vi "PiezoAndSnapshot.vi"() -> ()   [LabVIEW 2013]
doc: "v4: Added NI DAQ board instead of LabJack\n\nv5: Modified autofocus routine. Changed to triangle wave - AUTOFOCUS DOES NOT WORK ANYMORE\n\nv6: Modified autofocus to work with Triangle Wave. Added Saved Image Number to Lab Jack String."
uses:
  <vilib>/Platform/TimedLoop/XDataNode/timing_clust.ctl
  <vilib>/Platform/TimedLoop/XDataNode/nitl_modes.ctl
  <vilib>/Platform/TimedLoop/XDataNode/wakeup.ctl
  <vilib>/event_ctls.llb/eventvkey.ctl
  <vilib>/DAQmx/read.llb/DAQmx Read (Analog 1D DBL NChan 1Samp).vi
  <vilib>/DAQmx/miscellaneous.llb/DAQmx Fill In Error Info.vi
  <vilib>/platform/TimedLoop/XDataNode/XDataNode.xnode
  <vilib>/Platform/TimedLoop/XDataNode/XDNodeRunTimeDep.lvlib
panel:
  out "Voltage offset":dbl
  in  "Micron offset":dbl
  out "Counter":string
  out "TiffPath":string
  in  "Snap?":bool
  out "Stage Y":i32=31604
  out "Stage X":i32=-158372
  out "TotalFramesHidden":i32=27980
  out "Saved Images Hidden":i32=786
  out "sCMOS Image":u16[][](graph)
  in  "ROI":T1={"Horizontal Offset"=424, "Vertical Offset"=558, "Horizontal Width"=1200, "Vertical Width"=600}
  in  "Exposure (ms)":dbl=5.0
  in  "Binning":u16(ring)=1 items=["1x1"=1, "2x2"=2, "4x4"=4]
  out "Written":string="\r\r---------------------  NEW FILE  ---------------------\rO:\\20141210\\BrainScanner20141210_124111\r\r12/10/2014 12:42 PM\rcalib1\n\r\r12/10/2014 12:42 PM\rcalib 2\n\r\r12/10/2014 12:43 PM\rcalib 3\n\r\r"
  in  "Comments":string
  out "User Comments  File":path=path "O:/20141210/Comments.txt"
  out "Quit Pushed?":bool=TRUE
  out "Camera Trigger":dbl=0.00885779825410911 format="%.6f"
  out "Camera Frame File":path=path "O:/20141210/BrainScanner20141210_124111/CameraFrameData.txt"
  out "FxnGen Sync":dbl=3.893227260535598 format="%.6f"
  out "Z Sensor":dbl=0.9636767585825825 format="%.6f"
  out "LabJack File":path=path "O:/20141210/BrainScanner20141210_124111/LabJackData.txt"
  out "Current Image":u16[][](array[numeric])
  out "FuncGen Voltage":dbl=0.9652874538141194 format="%.6f"
  out "Z-ramp DC Offset":dbl=1.0
  out "sCMOS Camera Image File":path=path "O:/20141210/BrainScanner20141210_124111/sCMOS_Frames_U16_1024x1024.dat"
  out "Save Directory":path=path "O:/20141210/BrainScanner20141210_124111"
  out "Camera Info":string="C11440-22C; S/N: 751007; 2.50.A"
  in  "Quit":bool
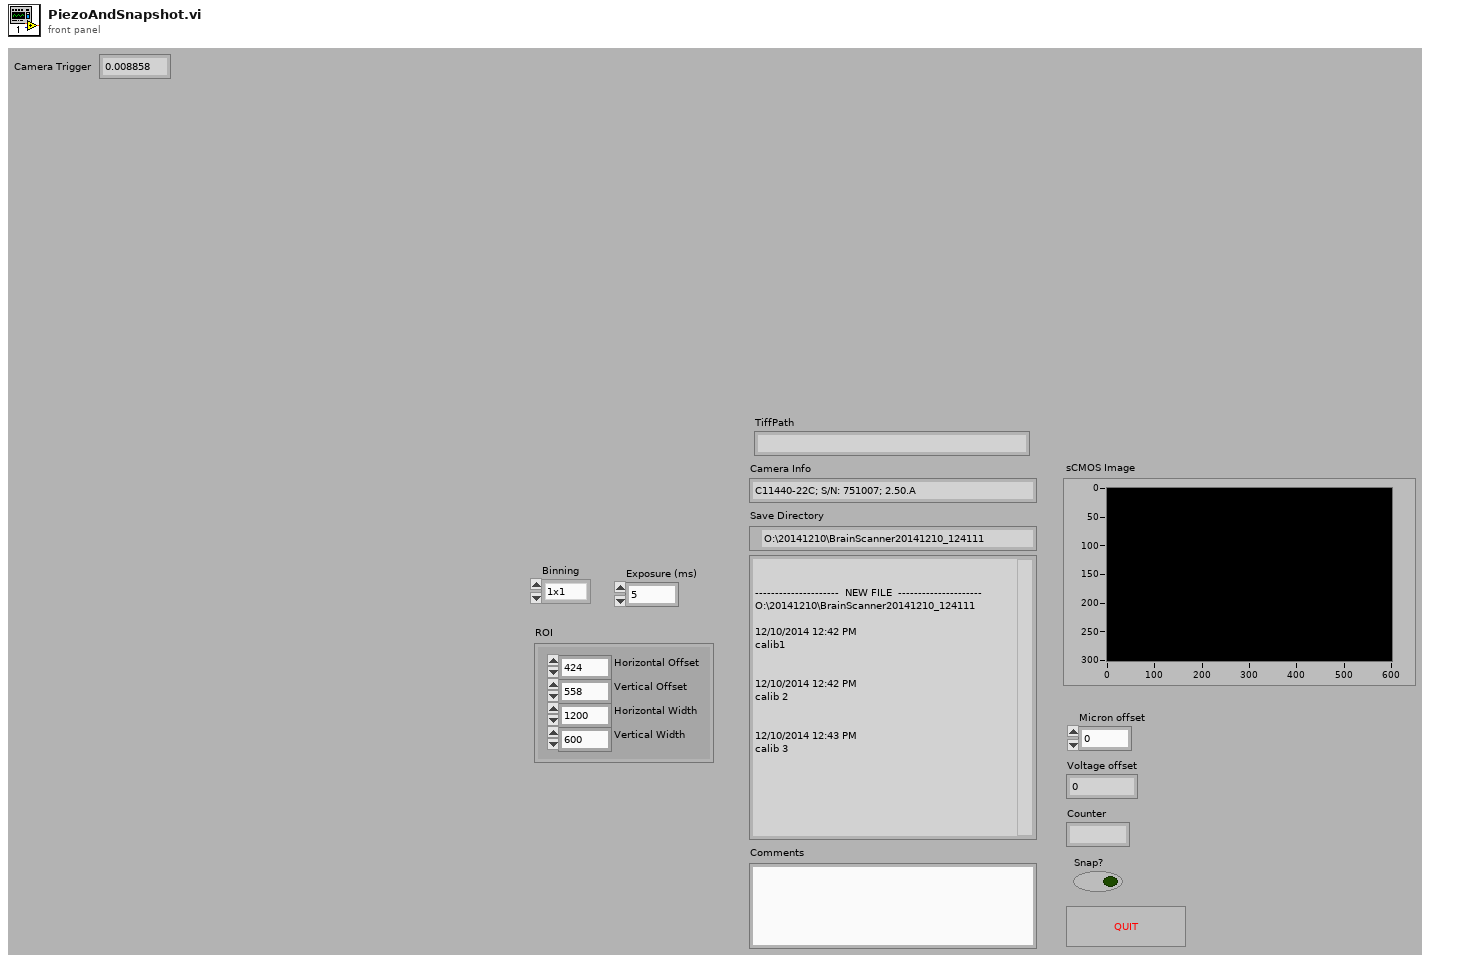
[diagram p1: front panel]
types:
  T1 = cluster{"Horizontal Offset":i32, "Vertical Offset":i32, "Horizontal Width":i32, "Vertical Width":i32}
  T2 = enum16{"open", "replace", "create", "open or create", "replace or create", "replace or create with confirmation"}
  T3 = cluster{"height":u32, "width":u32, "datatype":u32}
  T4 = cluster{"Mode":u32, "Polarity":u32, "Period":dbl, "Delay":dbl}
  T5 = typedef "XDNodeRunTimeDep.lvlib/timing_clust.ctl" = cluster{"Expected End [f-1]":u64, "Actual End [f-1]":u64, "Finished Late? [f-1]":bool, "Expected End [i-1]":u64, "Actual End [i-1]":u64, "Finished Late? [i-1]":bool, "Expected Start [i]":u64, "Actual Start [i]":u64, "Expected Start [f]":u64, "Actual Start [f]":u64, "Source Name":string, "Structure Name":string, "Period":i64, "Deadline":i64, "Offset":i64, "Start":i64, "Priority":i32, "Timeout":i32, "Mode":T6, "Wakeup Reason":T7, "Error":errorcluster, "Source Type":string, "Secondary Source Type":string, "Global End Time":u64, "Global Start Time":u64, "Frame Duration":u64, "Iteration Duration":u64, "Assigned CPU":i32, "I/O Scan Engine Mode":u32}
  T6 = typedef "XDNodeRunTimeDep.lvlib/nitl_modes.ctl" = enum32{"No Change", "Process missed periods, maintain original phase", "Discard missed periods, maintain original phase", "Process missed periods, ignore original phase", "Discard missed periods, ignore original phase"}
  T7 = typedef "XDNodeRunTimeDep.lvlib/wakeup.ctl" = enum32{"Normal", "Aborted", "Asynchronous wakeup", "Timing source error", "Timed loop error", "Timeout"}
  T8 = typedef "eventvkey.ctl" = enum16{"ASCII", "Enter", "Return", "Shift", "Ctrl", "Alt", "Cmd", "Opt", "Caps", "NumLock", "Clear", "Break", "Up", "Down", "Left", "Right", "Insert", "Delete", "Home", "End", "PageUp", "PageDown", "Escape", "Help", "Pause", "ScrollLock", "F1", "F2", "F3", "F4", "F5", "F6", "F7", "F8", "F9", "F10", "F11", "F12", "F13", "F14", "F15", "F16", "F17", "F18", "F19", "F20", "F21", "F22", "F23", "F24", "Play", "VolumeUp", "VolumeDown", "Mute", "Two Byte Char"}
  T9 = typedef "IMAQ Image.ctl" = refnum<image>
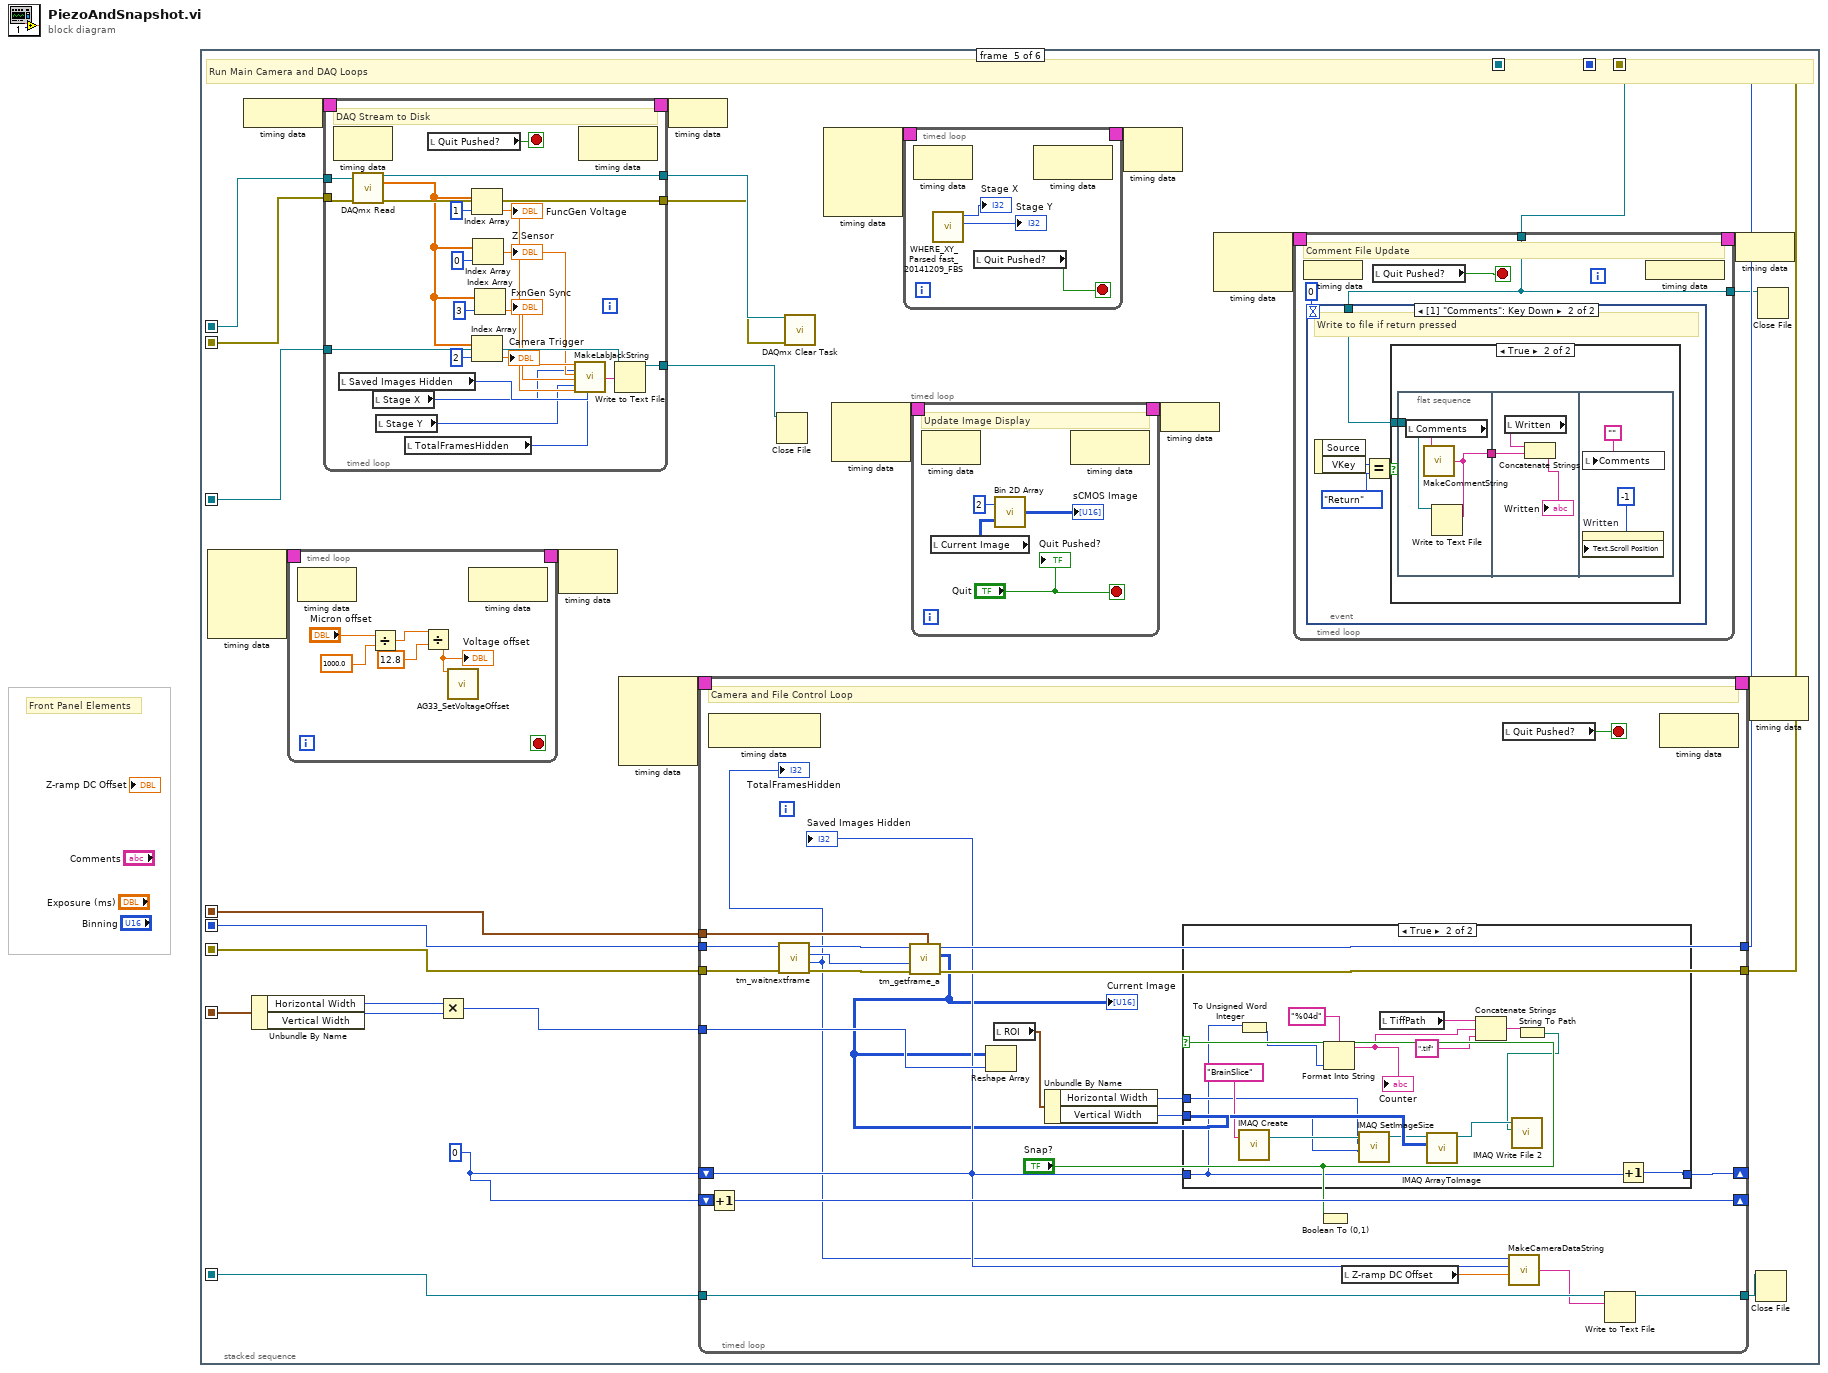
[diagram p0: block diagram]
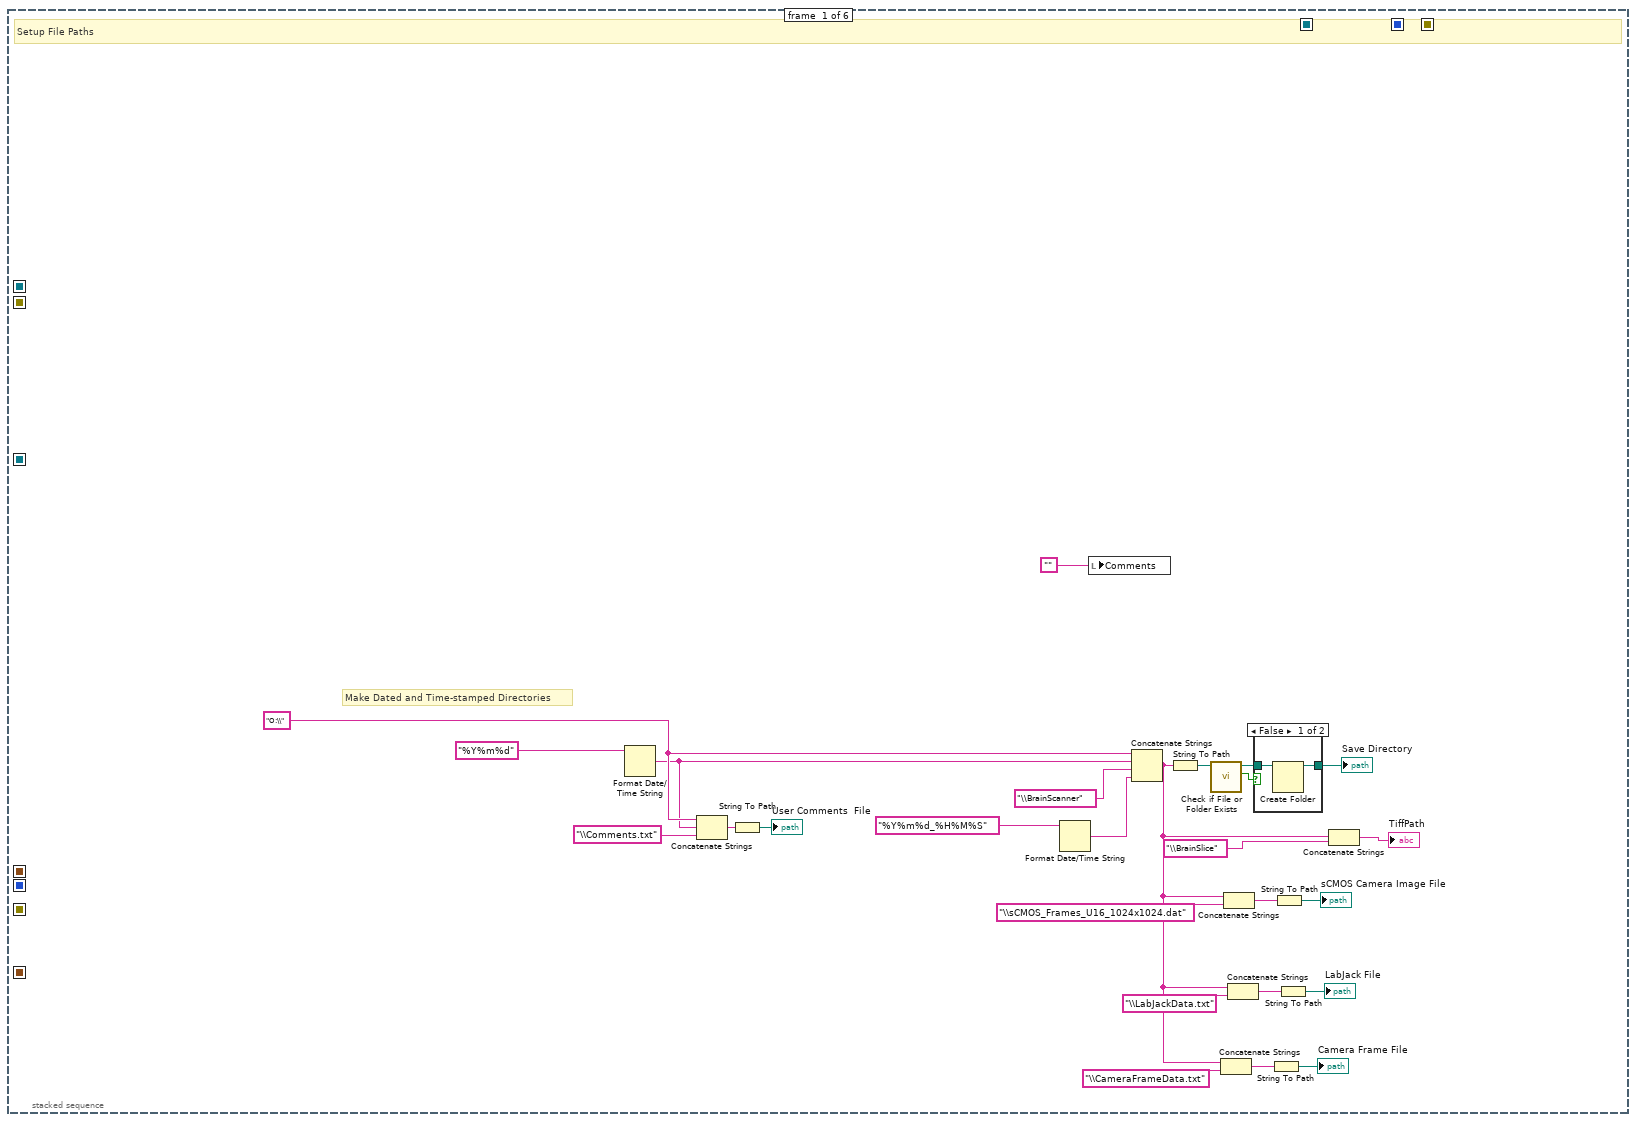
[diagram p2: hidden frame]
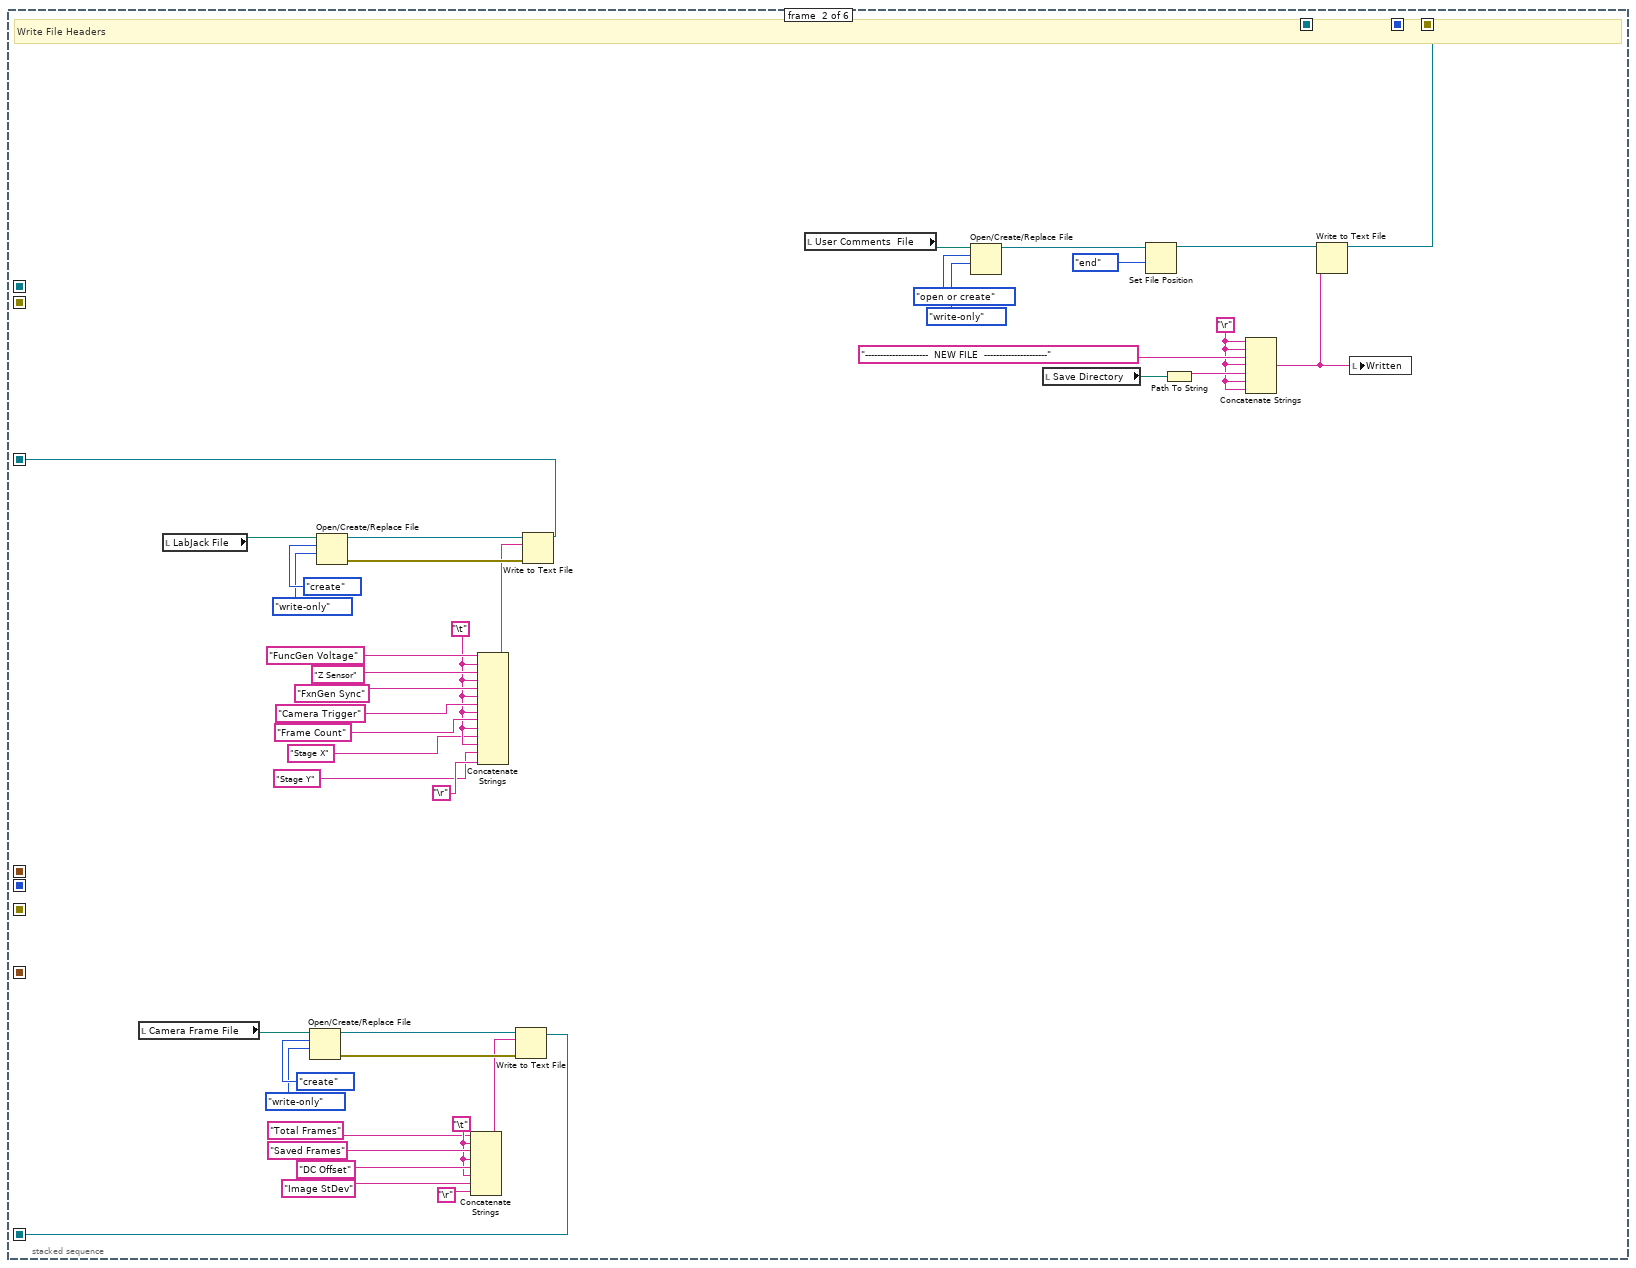
[diagram p4: hidden frame]
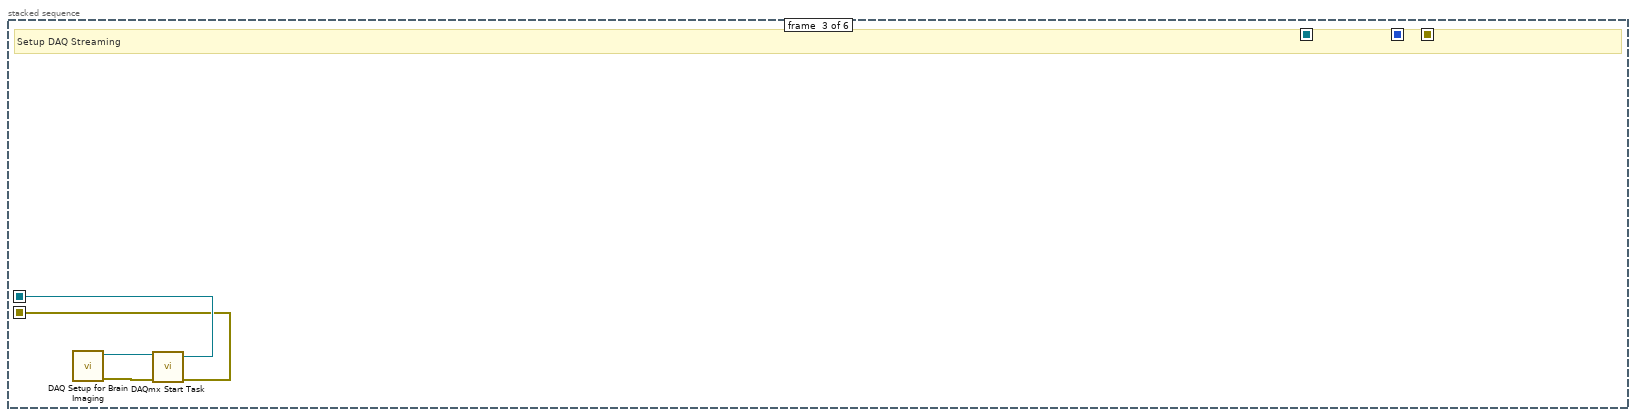
[diagram p5: hidden frame]
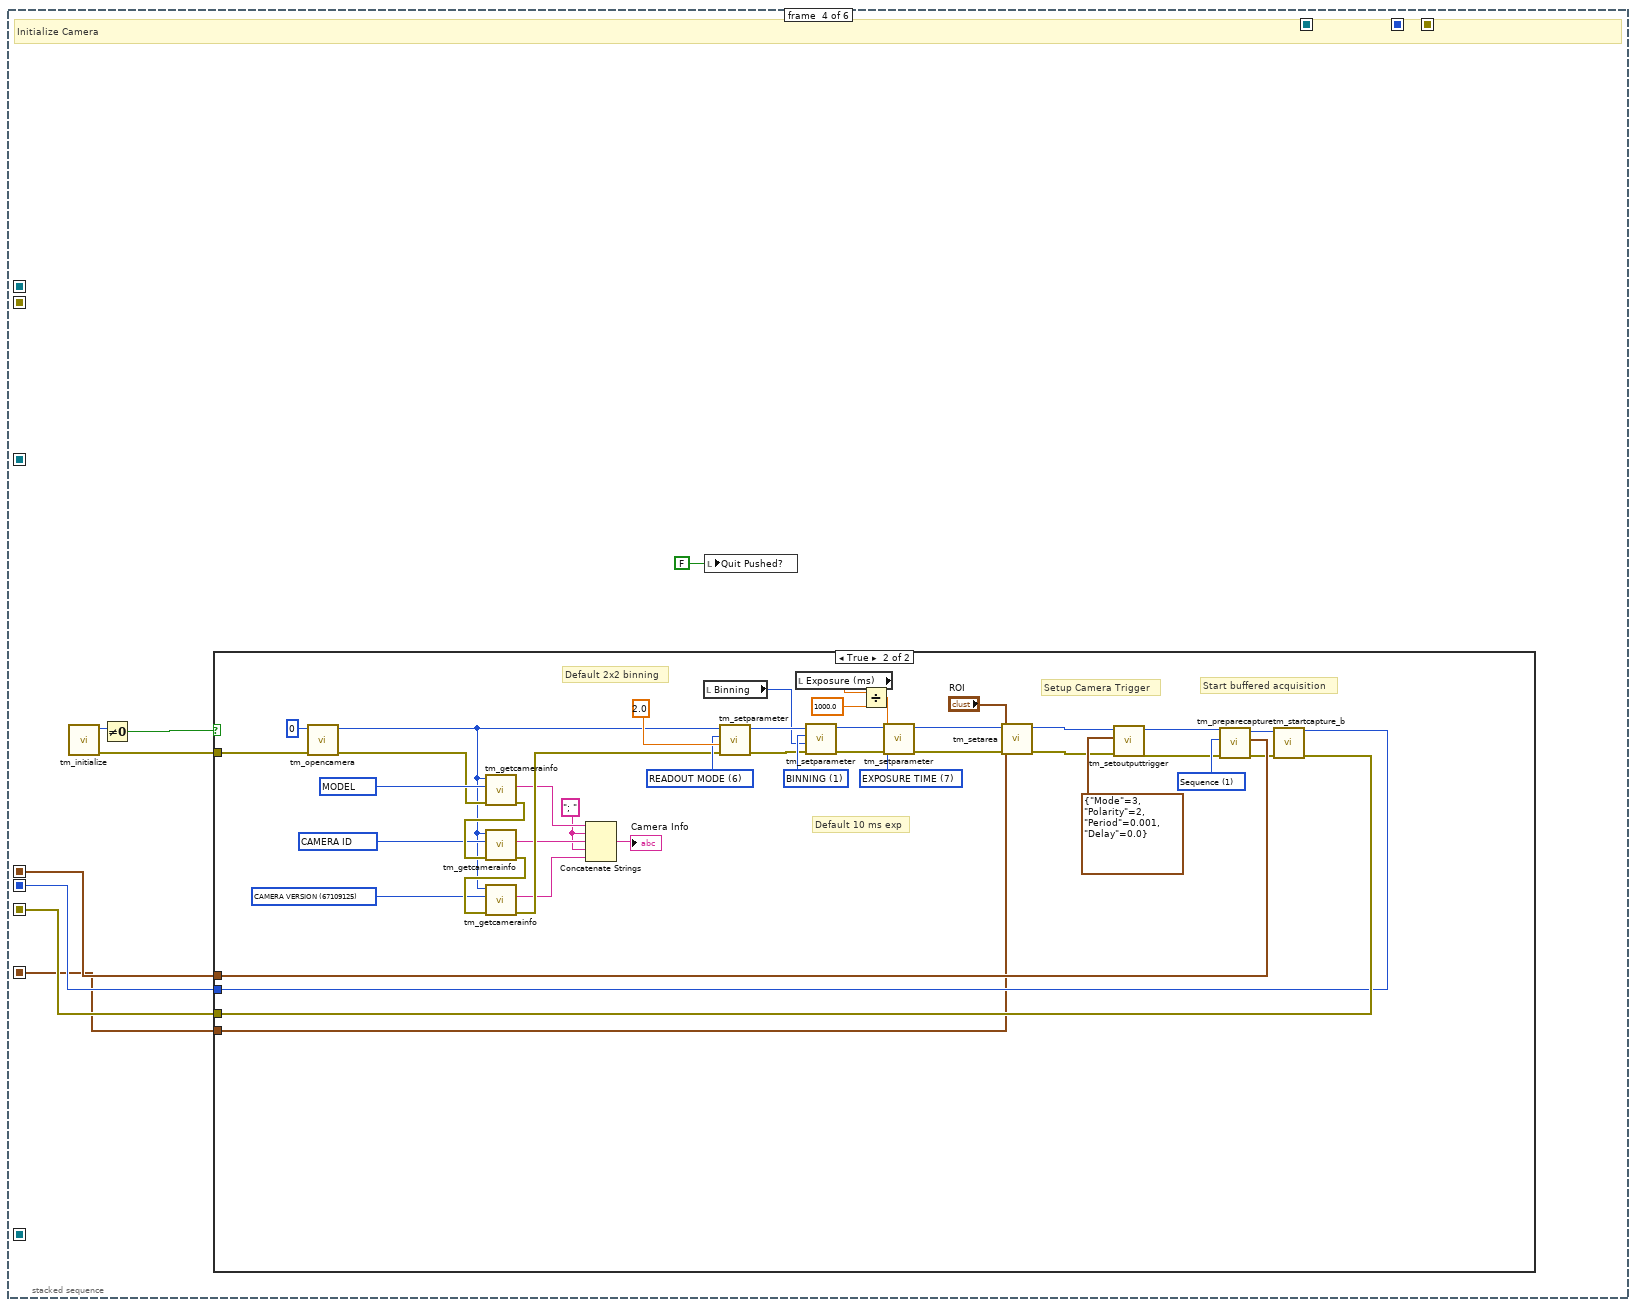
[diagram p6: hidden frame]
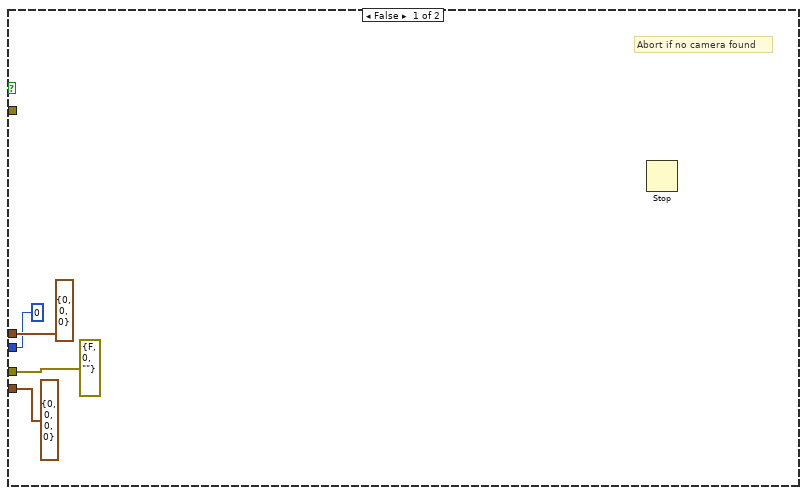
[diagram p7: hidden frame]
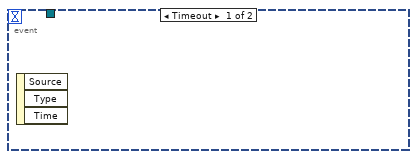
[diagram p8: hidden frame]
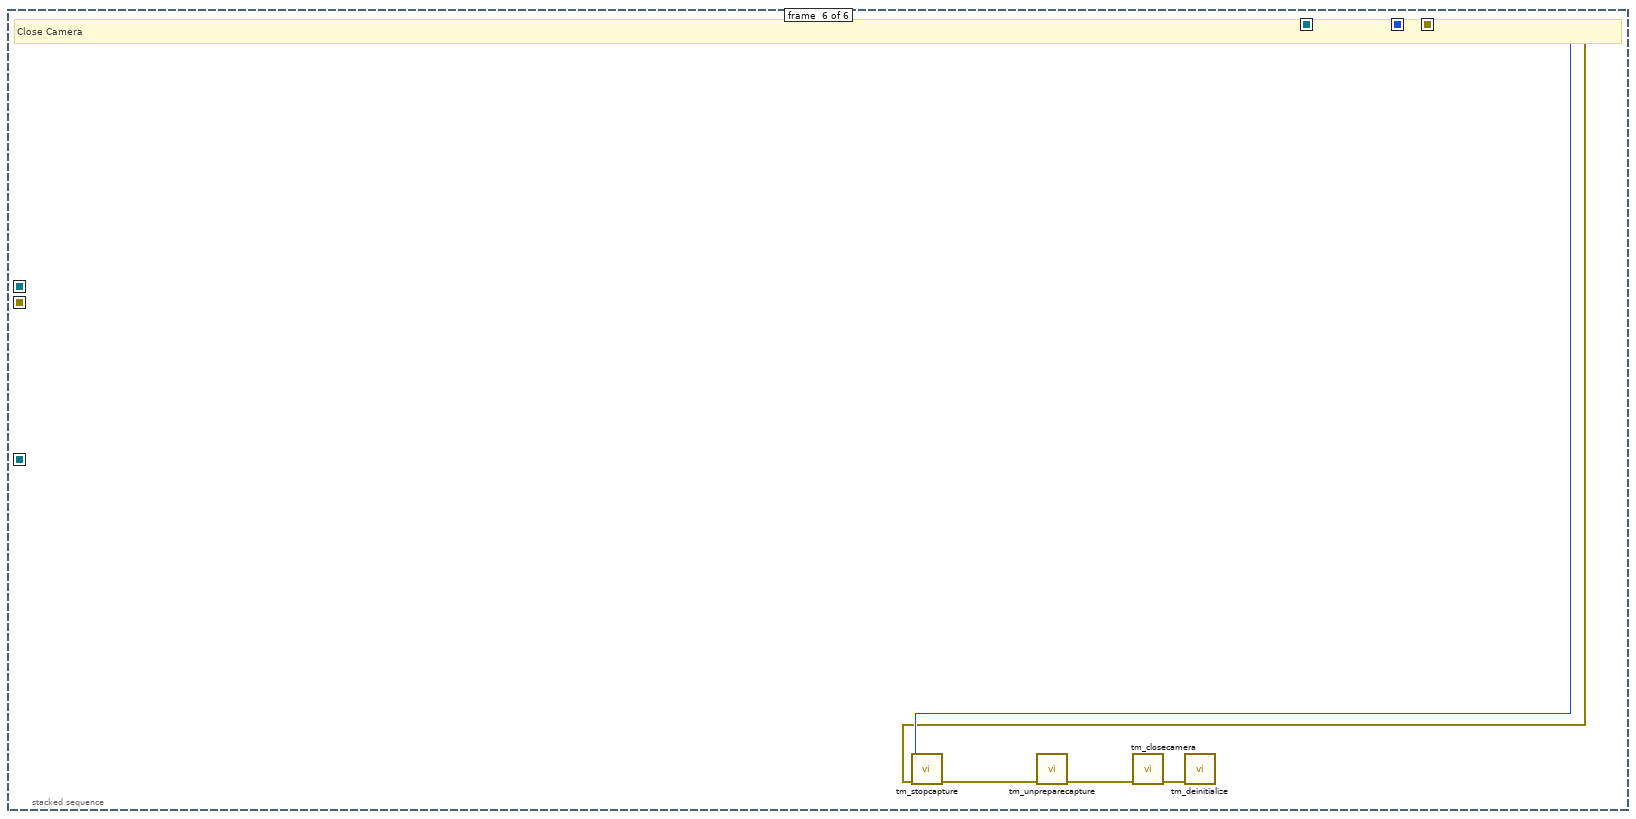
[diagram p11: hidden frame]
diagram:
  # "Front Panel Elements"
  n1 = stacked-sequence {
    seq-local: [_ _ _ w77 _ _] -> [_ _ _ _ w156 _]
    seq-local: [_ _ _ w78 _ _] -> [_ _ _ _ w159 _]
    seq-local: [_ _ _ w79 _ _] -> [_ _ _ _ w155 _]
    seq-local: [_ _ _ _ w158 _] -> [_ _ _ _ _ w276]
    seq-local: [_ _ _ _ w157 _] -> [_ _ _ _ _ w275]
    seq-local: [_ w64 _ _ _ _] -> [_ _ _ _ w147 _]
    seq-local: [_ _ w74 _ _ _] -> [_ _ _ _ w145 _]
    seq-local: [_ _ w73 _ _ _] -> [_ _ _ _ w146 _]
    seq-local: [_ w54 _ _ _ _] -> [_ _ _ _ w144 _]
    seq-local: [_ w42 _ _ _ _] -> [_ _ _ _ w140 _]
    seq-local: [_ _ _ w75 _ _] -> [_ _ _ _ w136 _]
    frame #0 {
      w7 = "O:\\"
      # "Make Dated and Time-stamped Directories"
      # "Setup File Paths"
      n2 = Format Date/Time String(time format string (%c)="%Y%m%d") -> (date/time string=w6:string)  [unwired: 2 in]
      n3 = Concatenate Strings(w7, w6, "\\Comments.txt" ("string")) -> (w4:string)
      n4 = String To Path(string=w4) -> (path=→"User Comments  File":path)
      n5 = Format Date/Time String(time format string (%c)="%Y%m%d_%H%M%S") -> (date/time string=w21:string)  [unwired: 2 in]
      n6 = local write "Comments"("") -> ()
      n7 = Concatenate Strings(w7, w6, "\\BrainScanner", w21) -> (w3:string)
      n8 = String To Path(string=w3) -> (path=w20:path)
      n9 = call <vilib>:"Check if File or Folder Exists.vi"("path"=w20) -> ("file or folder exists?"=w25:bool, "dup path"=w24:path)  [unwired: 8 in, 1 out]
      n10 = Concatenate Strings(w3, "\\CameraFrameData.txt" ("string")) -> (w12:string)
      n11 = Concatenate Strings(w3, "\\sCMOS_Frames_U16_1024x1024.dat" ("string")) -> (w17:string)
      n12 = Concatenate Strings(w3, "\\LabJackData.txt" ("string")) -> (w15:string)
      n13 = case shown="False" w25 {
        tunnel: [w27 w29] -> w19
        tunnel: w24 -> [w28 w29]
        frame False {
          n14 = Create Folder(path (use dialog)=w28) -> (created path=w27:path)  [unwired: 2 in, 2 out]
        }
        frame True {
        }
      }
      "Save Directory" <- w19
      n15 = String To Path(string=w12) -> (path=→"Camera Frame File":path)
      n16 = String To Path(string=w17) -> (path=→"sCMOS Camera Image File":path)
      n17 = String To Path(string=w15) -> (path=→"LabJack File":path)
      n18 = Concatenate Strings(w3, "\\BrainSlice" ("string")) -> (→"TiffPath":string)
    }
    frame #1 {
      w37 = "\r"
      w36 = "\t"
      w33 = "\t"
      # "Write File Headers"
      n19 = local read "Camera Frame File"() -> (w53:path)
      n20 = local read "LabJack File"() -> (w65:path)
      n21 = Open/Create/Replace File(file path (use dialog)=w53, operation (0:open)=T2."create", access (0:read/write)=enum16{"read/write", "read-only", "write-only"}."write-only") -> (refnum out=w63:refnum<file>, error out=w62:errorcluster)  [unwired: 3 in, 1 out]
      n22 = Open/Create/Replace File(file path (use dialog)=w65, operation (0:open)=T2."create", access (0:read/write)=enum16{"read/write", "read-only", "write-only"}."write-only") -> (refnum out=w70:refnum<file>, error out=w69:errorcluster)  [unwired: 3 in, 1 out]
      n23 = Concatenate Strings("Total Frames", w36, "Saved Frames", w36, "DC Offset", w36, "Image StDev", "\r") -> (w58:string)
      n24 = Concatenate Strings("FuncGen Voltage", w33, "Z Sensor", w33, "FxnGen Sync", w33, "Camera Trigger", w33, "Frame Count", w33, "Stage X" ("string"), w33, "Stage Y" ("string"), "\r") -> (w68:string)
      n25 = Write to Text File(file (use dialog)=w63, text=w58, error in=w62) -> (refnum out=w54:refnum<file>)  [unwired: 1 in, 2 out]
      n26 = Write to Text File(file (use dialog)=w70, text=w68, error in=w69) -> (refnum out=w64:refnum<file>)  [unwired: 1 in, 2 out]
      n27 = local read "User Comments  File"() -> (w48:path)
      n28 = Open/Create/Replace File(file path (use dialog)=w48, operation (0:open)=T2."open or create", access (0:read/write)=enum16{"read/write", "read-only", "write-only"}."write-only") -> (refnum out=w45:refnum<file>)  [unwired: 3 in, 2 out]
      n29 = local read "Save Directory"() -> (w40:path)
      n30 = Set File Position(refnum=w45, from (0:start)=enum16{"start", "end", "current"}."end") -> (refnum out=w43:refnum<file>)  [unwired: 2 in, 1 out]
      n31 = Path To String(path=w40) -> (string=w39:string)
      n32 = Concatenate Strings(w37, w37, "---------------------  NEW FILE  ---------------------", w37, w39, w37, w37) -> (w38:string)
      n33 = Write to Text File(file (use dialog)=w43, text=w38) -> (refnum out=w42:refnum<file>)  [unwired: 2 in, 2 out]
      n34 = local write "Written"(w38) -> ()
    }
    frame #2 {
      # "Setup DAQ Streaming"
      n35 = call "DAQ Setup for Brain Imaging.vi"() -> ("error out"=w71:errorcluster, "task out"=w72:refnum<k21>)  [unwired: 10 in]
      n36 = call <vilib>:"DAQmx Start Task.vi"("task/channels in"=w72, "error in"=w71) -> ("task out"=w74:refnum<k21>, "error out"=w73:errorcluster)  [unwired: 12 in]
    }
    frame #3 {
      # "Initialize Camera"
      n37 = call <userlib>:"tm_initialize.vi"() -> ("error out"=w82:errorcluster, "Number Of Cameras"=w80:u32)  [unwired: 10 in]
      n38 = Not Equal To 0?(x=w80) -> (x != 0?=w81:bool)
      n39 = case shown="True" w81 {
        tunnel: w82 -> [_ w127]
        tunnel: [errorcluster {"status"=FALSE, "code"=0, "source"=""} ("error out") w95] -> w79
        tunnel: [u32 0 ("Handle out") w94] -> w77
        tunnel: [T3 {"height"=0, "width"=0, "datatype"=0} ("Buffer Info") w116] -> w78
        tunnel: [T1 {"Horizontal Offset"=0, "Vertical Offset"=0, "Horizontal Width"=0, "Vertical Width"=0} ("ROI") "ROI"] -> w75
        frame False {
          # "Abort if no camera found"
          n40 = Stop() -> ()  [unwired: 1 in]
        }
        frame True {
          w100 = "; " ("string")
          w114 = u32 6 items=["BINNING"=1, "BITS PER CHANNEL"=2, "ACTIVE VIEW INDEX"=3, "CCD MODE"=4, "SENSOR MODE"=5, "READOUT MODE"=6, "EXPOSURE TIME"=7, "CONTRAST GAIN"=8, "CONTRAST OFFSET"=9, "LIGHT MODE"=10, "SENSITIVITY"=11, "WHITE BALANCE"=12, "PHOTON IMAGING MODE"=13, "HIGH DYNAMIC RANGE MODE"=14, "TRIGGER SOURCE"=15, "TRIGGER ACTIVE"=16, "TRIGGER MODE"=17, "TRIGGER POLARITY"=18, "TRIGGER GLOBAL EXPOSURE"=19, "FIRST TRIGGER BEHAVIOR"=20, "TRIGGER TIMES"=21, "OUTPUT TRIGGER POLARITY"=22, "OUTPUT TRIGGER DELAY"=23, "OUTPUT TRIGGER PERIOD"=24, "TEMPERATURE"=25, "TEMPERATURE TARGET"=26, "SENSOR COOLER FAN"=27, "MECHANICAL SHUTTER"=28, "BACK FOCUS POSITION"=29, "FRAMEBUNDLE MODE"=30, "FRAMEBUNDLE NUMBER"=31, "LINEBUNDLE HEIGHT"=32, "TRIGGER CONNECTOR"=33, "IMAGE PIXEL TYPE"=34, "OUTPUT TRIGGER KIND"=35, "READOUT DIRECTION"=36, "CHANNEL SYNC"=37] ("Parameter")
          w117 = 1 items=["Snap", "Sequence"] ("Capture mode")
          w118 = u32 7 items=["BINNING"=1, "BITS PER CHANNEL"=2, "ACTIVE VIEW INDEX"=3, "CCD MODE"=4, "SENSOR MODE"=5, "READOUT MODE"=6, "EXPOSURE TIME"=7, "CONTRAST GAIN"=8, "CONTRAST OFFSET"=9, "LIGHT MODE"=10, "SENSITIVITY"=11, "WHITE BALANCE"=12, "PHOTON IMAGING MODE"=13, "HIGH DYNAMIC RANGE MODE"=14, "TRIGGER SOURCE"=15, "TRIGGER ACTIVE"=16, "TRIGGER MODE"=17, "TRIGGER POLARITY"=18, "TRIGGER GLOBAL EXPOSURE"=19, "FIRST TRIGGER BEHAVIOR"=20, "TRIGGER TIMES"=21, "OUTPUT TRIGGER POLARITY"=22, "OUTPUT TRIGGER DELAY"=23, "OUTPUT TRIGGER PERIOD"=24, "TEMPERATURE"=25, "TEMPERATURE TARGET"=26, "SENSOR COOLER FAN"=27, "MECHANICAL SHUTTER"=28, "BACK FOCUS POSITION"=29, "FRAMEBUNDLE MODE"=30, "FRAMEBUNDLE NUMBER"=31, "LINEBUNDLE HEIGHT"=32, "TRIGGER CONNECTOR"=33, "IMAGE PIXEL TYPE"=34, "OUTPUT TRIGGER KIND"=35, "READOUT DIRECTION"=36, "CHANNEL SYNC"=37] ("Parameter")
          w119 = u32 1 items=["BINNING"=1, "BITS PER CHANNEL"=2, "ACTIVE VIEW INDEX"=3, "CCD MODE"=4, "SENSOR MODE"=5, "READOUT MODE"=6, "EXPOSURE TIME"=7, "CONTRAST GAIN"=8, "CONTRAST OFFSET"=9, "LIGHT MODE"=10, "SENSITIVITY"=11, "WHITE BALANCE"=12, "PHOTON IMAGING MODE"=13, "HIGH DYNAMIC RANGE MODE"=14, "TRIGGER SOURCE"=15, "TRIGGER ACTIVE"=16, "TRIGGER MODE"=17, "TRIGGER POLARITY"=18, "TRIGGER GLOBAL EXPOSURE"=19, "FIRST TRIGGER BEHAVIOR"=20, "TRIGGER TIMES"=21, "OUTPUT TRIGGER POLARITY"=22, "OUTPUT TRIGGER DELAY"=23, "OUTPUT TRIGGER PERIOD"=24, "TEMPERATURE"=25, "TEMPERATURE TARGET"=26, "SENSOR COOLER FAN"=27, "MECHANICAL SHUTTER"=28, "BACK FOCUS POSITION"=29, "FRAMEBUNDLE MODE"=30, "FRAMEBUNDLE NUMBER"=31, "LINEBUNDLE HEIGHT"=32, "TRIGGER CONNECTOR"=33, "IMAGE PIXEL TYPE"=34, "OUTPUT TRIGGER KIND"=35, "READOUT DIRECTION"=36, "CHANNEL SYNC"=37] ("Parameter")
          w120 = u32 67109122 items=["BUS"=67109121, "CAMERA ID"=67109122, "VENDOR"=67109123, "MODEL"=67109124, "CAMERA VERSION"=67109125, "DRIVER VERSION"=67109126, "MODULE VERSIOIN"=67109127, "DCAMAPI VERSION"=67109128] ("Info ID")
          w122 = u32 67109125 items=["BUS"=67109121, "CAMERA"=67109122, "VENDOR"=67109123, "MODEL"=67109124, "CAMERA VERSION"=67109125, "DRIVER VERSION"=67109126, "MODULE VERSIOIN"=67109127, "DCAMAPI VERSION"=67109128] ("Info ID")
          w125 = u32 67109124 items=["BUS"=67109121, "CAMERA"=67109122, "VENDOR"=67109123, "MODEL"=67109124, "CAMERA VERSION"=67109125, "DRIVER VERSION"=67109126, "MODULE VERSIOIN"=67109127, "DCAMAPI VERSION"=67109128] ("Info ID")
          # "Start buffered acquisition"
          # "Setup Camera Trigger"
          # "Default 10 ms exp"
          # "Default 2x2 binning"
          n41 = call <userlib>:"tm_opencamera.vi"("error in (no error)"=w127, "Camera Index"=u32 0) -> ("error out"=w121:errorcluster, "Handle out"=w106:u32)  [unwired: 8 in]
          n42 = call <userlib>:"tm_getcamerainfo.vi"("error in (no error)"=w121, "Info ID"=w125, "Handle in"=w106) -> ("error out"=w124:errorcluster, "String"=w103:string)  [unwired: 6 in, 1 out]
          n43 = call <userlib>:"tm_getcamerainfo.vi"("error in (no error)"=w124, "Info ID"=w120, "Handle in"=w106) -> ("error out"=w123:errorcluster, "String"=w102:string)  [unwired: 6 in, 1 out]
          n44 = call <userlib>:"tm_getcamerainfo.vi"("error in (no error)"=w123, "Info ID"=w122, "Handle in"=w106) -> ("error out"=w105:errorcluster, "String"=w101:string)  [unwired: 6 in, 1 out]
          n45 = Concatenate Strings(w103, w100, w102, w100, w101) -> (→"Camera Info":string)
          n46 = local read "Binning"() -> (w97:u16)
          n47 = call <userlib>:"tm_setparameter.vi"("error in (no error)"=w105, "Value in"=2.0, "Parameter"=w114, "Handle in"=w106) -> ("error out"=w107:errorcluster, "Handle out"=w108:u32)  [unwired: 6 in]
          n48 = local read "Exposure (ms)"() -> (w96:dbl)
          n49 = call <userlib>:"tm_setparameter.vi"("error in (no error)"=w107, "Value in"=w97, "Parameter"=w119, "Handle in"=w108) -> ("error out"=w112:errorcluster, "Handle out"=w113:u32)  [unwired: 6 in]
          n50 = Divide(x=w96, y=1000.0) -> (x/y=w98:dbl)
          n51 = call <userlib>:"tm_setparameter.vi"("error in (no error)"=w112, "Value in"=w98, "Parameter"=w118, "Handle in"=w113) -> ("error out"=w93:errorcluster, "Handle out"=w92:u32)  [unwired: 6 in]
          n52 = call <userlib>:"tm_setarea.vi"("error in (no error)"=w93, "Sub Region"="ROI", "Handle in"=w92) -> ("error out"=w90:errorcluster, "Handle out"=w91:u32)  [unwired: 7 in]
          n53 = call <userlib>:"tm_setoutputtrigger.vi"("error in (no error)"=w90, "Parameters"=T4 {"Mode"=3, "Polarity"=2, "Period"=0.001, "Delay"=0.0}, "Handle in"=w91) -> ("error out"=w88:errorcluster, "Handle out"=w89:u32)  [unwired: 7 in]
          n54 = call <userlib>:"tm_preparecapture.vi"("error in (no error)"=w88, "Capture mode"=w117, "Handle in"=w89) -> ("error out"=w110:errorcluster, "Buffer Info"=w116:T3, "Handle out"=w111:u32)  [unwired: 5 in, 1 out]
          n55 = call <userlib>:"tm_startcapture_b.vi"("error in (no error)"=w110, "Handle in"=w111) -> ("error out"=w95:errorcluster, "Handle out"=w94:u32)  [unwired: 8 in]
        }
      }
      n56 = local write "Quit Pushed?"(FALSE ("stop")) -> ()
    }
    frame #4 {
      w138 = 0
      # "Run Main Camera and DAQ Loops"
      n57 = node-c288() -> (w129:T5)  [unwired: 4 in]
      n58 = node-c288() -> (w152:T5)
      n59 = Unbundle By Name(w136) -> ("Horizontal Width"=w135:i32, "Vertical Width"=w134:i32)
      n60 = timed-loop {
        timing: w129 -> [_]
        timing-out: [_] -> w128
        stop <- _ stop-if-true
        n61 = node-c288() -> ()  [unwired: 1 in, 1 out]
        n62 = Divide(x="Micron offset", y=1000.0) -> (x/y=w161:dbl)
        n63 = Divide(x=w161, y=12.8) -> (x/y=w162:dbl)
        "Voltage offset" <- w162
        n64 = call "AG33_SetVoltageOffset.vi"("DC Offset (0.00 V)"=w162) -> ()  [unwired: 2 in, 1 out]
        n65 = node-c288() -> ()  [unwired: 1 in, 1 out]
      }
      n66 = timed-loop {
        timing: w152 -> [_]
        timing-out: [_] -> w151
        tunnel: w145 -> [w214]
        tunnel: w146 -> [w213]
        tunnel: [w221] -> w150
        tunnel: w147 -> [w220]
        tunnel: [w212] -> w133
        tunnel: [w211] -> w132
        stop <- w215 stop-if-true
        # "DAQ Stream to Disk"
        n67 = node-c288() -> ()  [unwired: 1 in, 1 out]
        n68 = local read "Saved Images Hidden"() -> (w208:i32)
        n69 = call-poly <vilib>:"DAQmx Read.vi"("task/channels in"=w214, "error in"=w213) -> ("task out"=w212:refnum<k21>, "data"=w210:dbl[], "error out"=w211:errorcluster)  [unwired: 11 in]
        n70 = local read "Stage X"() -> (w206:i32)
        n71 = local read "Stage Y"() -> (w205:i32)
        n72 = local read "TotalFramesHidden"() -> (w207:i32)
        n73 = local read "Quit Pushed?"() -> (w215:bool)
        n74 = Index Array(array=w210, index=1 ("index (row)")) -> (element=w219:dbl)
        "FuncGen Voltage" <- w219
        n75 = Index Array(array=w210, index=2 ("index (row)")) -> (element=w216:dbl)
        "Camera Trigger" <- w216
        n76 = Index Array(array=w210, index=0 ("index (row)")) -> (element=w218:dbl)
        "Z Sensor" <- w218
        n77 = Index Array(array=w210, index=3 ("index (row)")) -> (element=w217:dbl)
        "FxnGen Sync" <- w217
        n78 = call "MakeLabJackString.vi"("FuncGen Voltage"=w219, "X position"=w206, "Z Sensor"=w218, "Photodiode"=w217, "Y position"=w205, "Camera Trigger"=w216, "Total Frame Count"=w207, "Save Image Counts"=w208) -> ("Output String"=w222:string)  [unwired: 11 in]
        n79 = node-c288() -> ()  [unwired: 1 in, 1 out]
        n80 = Write to Text File(file (use dialog)=w220, text=w222) -> (refnum out=w221:refnum<file>)  [unwired: 2 in, 2 out]
      }
      n81 = Multiply(x=w135, y=w134) -> (x*y=w137:i32)
      n82 = node-c288(w128) -> ()  [unwired: 1 out]
      n83 = node-c288() -> (w154:T5)  [unwired: 4 in]
      n84 = node-c288(w151) -> ()
      n85 = timed-loop "Timed Loop" {
        tunnel: w155 -> [w252]
        tunnel: [w251] -> w158
        tunnel: [w250] -> w157
        tunnel: w156 -> [w253]
        shift-right: [w239] -> _
        shift-left: w138 -> [w236]
        timing: w154 -> [_]
        timing-out: [_] -> w153
        tunnel: w159 -> [w249]
        tunnel: w144 -> [w245]
        tunnel: [w244] -> w143
        shift-right: [w238] -> _
        shift-left: w138 -> [w240]
        tunnel: w137 -> [w237]
        stop <- w241 stop-if-true
        # "Camera and File Control Loop"
        n86 = node-c288() -> ()  [unwired: 1 in, 1 out]
        n87 = Increment(x=w240) -> (x+1=w238:i32)
        n88 = call <userlib>:"tm_waitnextframe.vi"("error in (no error)"=w252, "Handle in"=w253) -> ("error out"=w248:errorcluster, "Frame Count"=w235:i32, "Frame Index"=w246:i32, "Handle out"=w247:u32)  [unwired: 6 in]
        "TotalFramesHidden" <- w235
        n89 = call <userlib>:"tm_getframe_a.vi"("error in (no error)"=w248, "Frame Index"=w246, "Buffer Info"=w249, "Handle in"=w247) -> ("error out"=w250:errorcluster, "Data 16"=w233:u16[][], "Handle out"=w251:u32)  [unwired: 3 in, 2 out]
        "Current Image" <- w233
        n90 = Reshape Array(w233, w237) -> ()  [unwired: 1 out]
        n91 = local read "ROI"() -> (w234:T1)
        n92 = Unbundle By Name(w234) -> ("Horizontal Width"=w231:i32, "Vertical Width"=w230:i32)
        n93 = case shown="True" "Snap?" {
          tunnel: w236 -> [w254 w255]
          tunnel: [w254 w270] -> w239
          tunnel: w233 -> [_ w269]
          tunnel: w231 -> [_ w266]
          tunnel: w230 -> [_ w265]
          frame False {
          }
          frame True {
            n94 = To Unsigned Word Integer(number=w255) -> (unsigned 16bit integer=w262:u16)
            n95 = call "IMAQ Create"("Image Name"="BrainSlice") -> ("New Image"=w268:T9)  [unwired: 4 in, 1 out]
            n96 = Format Into String(format string="%04d", w262) -> (resulting string=w260:string)  [unwired: 2 in, 1 out]
            "Counter" <- w260
            n97 = call "IMAQ SetImageSize"("Y Resolution"=w265, "X Resolution"=w266, "Image"=w268) -> ("Image Out"=w263:T9)  [unwired: 2 in, 1 out]
            n98 = local read "TiffPath"() -> (w261:string)
            n99 = call "IMAQ ArrayToImage"("Image Pixels (U8)"=w269, "Image"=w263) -> ("Image Out"=w264:T9)  [unwired: 8 in, 1 out]
            n100 = Concatenate Strings(w261, w260, ".tif" ("string")) -> (w258:string)
            n101 = String To Path(string=w258) -> (path=w257:path)
            n102 = call-poly "IMAQ Write File 2"("File Path"=w257, "Image"=w264) -> ()  [unwired: 8 in, 2 out]
            n103 = Increment(x=w255) -> (x+1=w270:i32)
          }
        }
        n104 = Boolean To (0,1)(Boolean="Snap?") -> ()  [unwired: 1 out]
        n105 = local read "Z-ramp DC Offset"() -> (w242:dbl)
        n106 = local read "Quit Pushed?"() -> (w241:bool)
        n107 = call "MakeCameraDataString.vi"("DC Offset"=w242, "Saved Frame Number"=w236, "Frame Number"=w235) -> ("Output String"=w243:string)  [unwired: 1 in]
        n108 = Write to Text File(file (use dialog)=w245, text=w243) -> (refnum out=w244:refnum<file>)  [unwired: 2 in, 2 out]
        n109 = node-c288() -> ()  [unwired: 1 in, 1 out]
        "Saved Images Hidden" <- w236
      }
      n110 = Close File(refnum=w150) -> ()  [unwired: 1 in, 2 out]
      n111 = call <vilib>:"DAQmx Clear Task.vi"("task in"=w133, "error in"=w132) -> ()  [unwired: 13 in, 1 out]
      n112 = node-c288() -> (w131:T5)  [unwired: 4 in]
      n113 = node-c288() -> (w149:T5)  [unwired: 2 in]
      n114 = timed-loop {
        timing: w131 -> [_]
        timing-out: [_] -> w130
        stop <- w171 stop-if-true
        n115 = node-c288() -> ()  [unwired: 1 in, 1 out]
        n116 = call "WHERE_XY_Parsed fast_20141209_FBS.vi"() -> ("X"=→"Stage X":i32, "Y"=→"Stage Y":i32)  [unwired: 1 in, 2 out]
        n117 = local read "Quit Pushed?"() -> (w171:bool)
        n118 = node-c288() -> ()  [unwired: 1 in, 1 out]
      }
      n119 = timed-loop {
        timing: w149 -> [_]
        timing-out: [_] -> w148
        stop <- "Quit" stop-if-true
        # "Update Image Display"
        n120 = node-c288() -> ()  [unwired: 1 in, 1 out]
        n121 = local read "Current Image"() -> (w198:u16[][])
        n122 = call "Bin 2D Array.vi"("Input Array"=w198, "Binning Value"=u8 2) -> ("Binned Array"=→"sCMOS Image":u16[][])
        n123 = node-c288() -> ()  [unwired: 1 in, 1 out]
        "Quit Pushed?" <- "Quit"
      }
      n124 = node-c288(w130) -> ()  [unwired: 1 out]
      n125 = node-c288(w148) -> ()
      n126 = node-c288() -> (w142:T5)  [unwired: 2 in]
      n127 = timed-loop {
        timing: w142 -> [_]
        timing-out: [_] -> w141
        tunnel: w140 -> [w177]
        tunnel: [w177] -> w139
        stop <- w178 stop-if-true
        # "Comment File Update"
        n128 = node-c288() -> ()  [unwired: 1 in]
        n129 = event shown="[1] \"Comments\": Key Down" {
          selector: _ -> [_ _]
          dyn-events: _ -> [_ _]
          timeout: 0 -> [_ _]
          tunnel: w177 -> [_ w179]
          event Timeout {
            n130 = event-data() -> ()  [unwired: 1 in, 3 out]
          }
          event "Comments": Key Down {
            # "Write to file if return pressed"
            n131 = event-data() -> ("VKey"=w182:T8)  [unwired: 1 in, 1 out]
            n132 = Equal?(x=w182, y=eventvkey."Return") -> (x = y?=w180:bool)
            n133 = case shown="True" w180 {
              tunnel: w179 -> [_ w184]
              frame False {
              }
              frame True {
                n134 = flat-sequence {
                  tunnel: w184 -> [w187]
                  tunnel: [w186] -> w183
                  tunnel: w183 -> [w189]
                  frame #0 {
                    n135 = local read "Comments"() -> (w185:string)
                    n136 = call "MakeCommentString.vi"("Input string"=w185) -> ("Output String"=w186:string)
                    n137 = Write to Text File(file (use dialog)=w187, text=w186) -> ()  [unwired: 2 in, 3 out]
                  }
                  frame #1 {
                    n138 = local read "Written"() -> (w190:string)
                    n139 = Concatenate Strings(w190, w189) -> (→"Written":string)
                  }
                  frame #2 {
                    n140 = local write "Comments"("") -> ()
                    n141 = property on="Written" class="Str"("Text.Scroll Position"=-1) -> ()  [unwired: 2 in, 2 out]
                  }
                }
              }
            }
          }
        }
        n142 = local read "Quit Pushed?"() -> (w178:bool)
        n143 = node-c288() -> ()  [unwired: 1 out]
      }
      n144 = node-c288(w141) -> ()
      n145 = node-c288 ("Output Node")(w153) -> ()  [unwired: 1 out]
      n146 = Close File(refnum=w143) -> ()  [unwired: 1 in, 2 out]
      n147 = Close File(refnum=w139) -> ()  [unwired: 1 in, 2 out]
    }
    frame #5 {
      # "Close Camera"
      n148 = call <userlib>:"tm_stopcapture.vi"("error in (no error)"=w275, "Handle in"=w276) -> ("error out"=w278:errorcluster)  [unwired: 8 in, 1 out]
      n149 = call <userlib>:"tm_unpreparecapture.vi"("error in (no error)"=w278) -> ("error out"=w277:errorcluster)  [unwired: 9 in, 1 out]
      n150 = call <userlib>:"tm_closecamera.vi"("error in (no error)"=w277) -> ("error out"=w279:errorcluster)  [unwired: 10 in]
      n151 = call <userlib>:"tm_deinitialize.vi"("error in (no error)"=w279) -> ()  [unwired: 10 in, 1 out]
    }
  }
